vi "Lock-in Command.vi"(6 "Context":T1, 8 "error in (no error)":errorcluster, 9 "Request type":T2=enum."User command", 10 "Lock-in":bool, 11 "Lockin Digitizer in":refnum<class "Lockin Digitizer.lvclass">) -> (0 "error out":errorcluster, 3 "Lockin Digitizer out":refnum<class "Lockin Digitizer.lvclass">, 4 "Result":refnum<class "Acquired Result.lvclass">)   [LabVIEW 2021, in "Lockin Digitizer.lvclass"]
uses:
  Lockin Digitizer.lvclass
  C:/GitHub/LabActor/Template Module/Template Module.lvclass
  NHMFL_Core/Libraries/Instruments/Results/Acquired Result/Acquired Result.lvclass
  Controllers/Process Controller/Request type.ctl
  L-D Command Context.ctl
  Worker/Worker Actor/Background Loop Action.ctl
  Template Module/Template Module.lvclass/Template Module.ctl
  NHMFL_Core/Libraries/Instruments/Instrument Driver/Instrument Driver.lvclass/Instrument Driver.ctl
  Template Module/Read Configuration.vi
  Template Module/Read Name.vi
  NHMFL_Core/Libraries/Instruments/Instrument Driver/Write Recorder name.vi
  NHMFL_Core/Libraries/Instruments/Pulse Driver/Lockin Digitizer Driver/Lockin Digitizer Driver.lvclass
  C:/GitHub/NHMFL_Core/Libraries/Instruments/Instrument Driver/Instrument Driver.lvclass
  NHMFL_Core/Libraries/Instruments/Instrument Driver/Write User configuration.vi
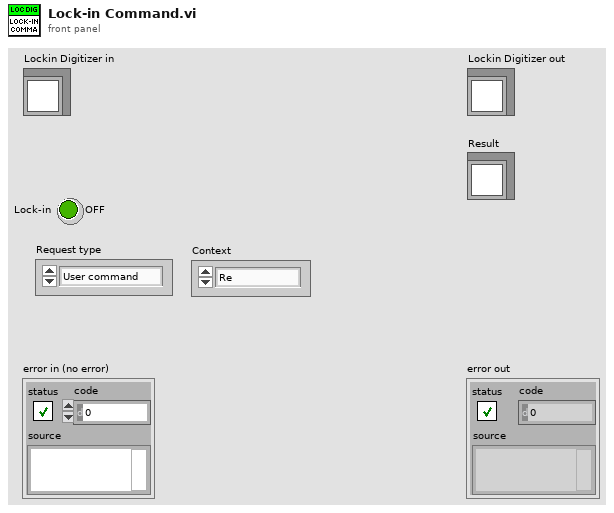
[diagram p1: front panel]
types:
  T1 = typedef "L-D Command Context.ctl" = enum16{"Re", "Switch", "Measure", "Arm"}
  T2 = typedef "Request type.ctl" = enum16{"Process complete", "User command", "Auto-restart", "Error"}
  T3 = typedef "Background Loop Action.ctl" = enum16{"Start", "Continue", "Stop"}
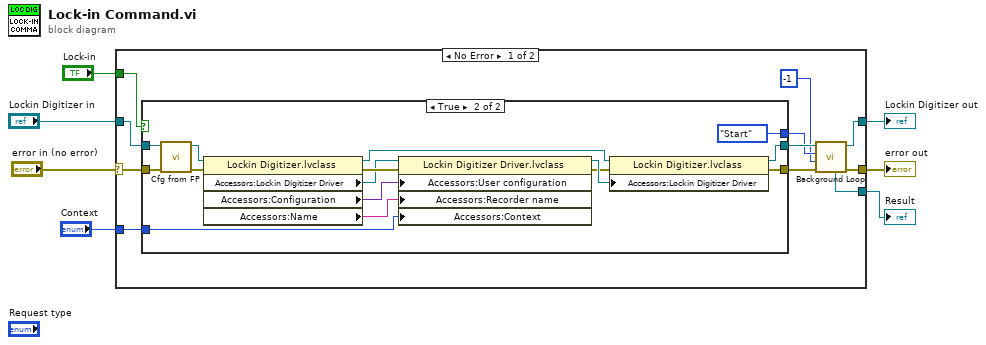
[diagram p0: block diagram]
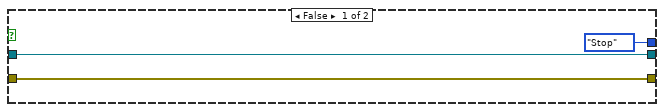
[diagram p2: hidden frame]
diagram:
  n1 = case shown="No Error" "error in (no error)" {
    selector: "error in (no error)" -> [w15 w38]
    tunnel: [w18 w38] -> w6
    tunnel: [w17 w37] -> w4
    tunnel: "Lockin Digitizer in" -> [w13 w37]
    tunnel: "Lock-in" -> [w16 _]
    tunnel: [w10 _] -> w2
    tunnel: "Context" -> [w8 _]
    frame No Error {
      n2 = case shown="True" w16 {
        tunnel: w13 -> [w20 w32]
        tunnel: w15 -> [w19 w29]
        tunnel: [w20 w25] -> w14
        tunnel: [Background_Loop_Action."Stop" ("Action") Background_Loop_Action."Start" ("Action")] -> w12
        tunnel: [w19 w23] -> w11
        tunnel: w8 -> [_ w22]
        frame False {
        }
        frame True {
          n3 = call-dynamic "Cfg from FP.vi"("error in (no error)"=w29, "Measure Object in"=w32) -> ("error out"=w30:errorcluster, "Measure Object out"=w31:refnum<class "Lockin Digitizer.lvclass">)  [unwired: 8 in]
          n4 = property class="Lockin Digitizer.lvclass"(reference=w31, error in=w30) -> (reference out=w27:refnum<class "Lockin Digitizer.lvclass">, error out=w34:errorcluster, "Accessors:Lockin Digitizer Driver"=w33:refnum<class "Lockin Digitizer Driver.lvclass">, "Accessors:Configuration"=w36:variant, "Accessors:Name"=w35:string)
          n5 = property class="Lockin Digitizer Driver.lvclass"(reference=w33, error in=w34, "Accessors:User configuration"=w36, "Accessors:Recorder name"=w35, "Accessors:Context"=w22) -> (reference out=w26:refnum<class "Lockin Digitizer Driver.lvclass">, error out=w24:errorcluster)
          n6 = property class="Lockin Digitizer.lvclass"(reference=w27, error in=w24, "Accessors:Lockin Digitizer Driver"=w26) -> (reference out=w25:refnum<class "Lockin Digitizer.lvclass">, error out=w23:errorcluster)
        }
      }
      n7 = call-dynamic "Background Loop.vi"("error in (no error)"=w11, "Loop number"=-1, "Action"=w12, "Worker in"=w14) -> ("error out"=w18:errorcluster, "Worker out"=w17:refnum<class "Lockin Digitizer.lvclass">, "Result"=w10:refnum<class "Acquired Result.lvclass">)  [unwired: 5 in]
    }
    frame Error {
    }
  }
  "error out" <- w6
  "Lockin Digitizer out" <- w4
  "Result" <- w2
